vi "Writer Listen.vi"(8 "error in (no error)":errorcluster, 11 "TCP Writer in":refnum<class "TCP Writer.lvclass">) -> (0 "error out":errorcluster, 3 "TCP Writer out":refnum<class "TCP Writer.lvclass">)   [LabVIEW 2018, in "TCP Classes.lvlib" / "TCP Writer.lvclass"]
uses:
  TCP Writer.lvclass
  C:/Users/Jeff Tipps/Documents/DAQMan/source/Classes/TCP Server/Class TCP Connection/TCP Connection.lvclass
  C:/Program Files (x86)/National Instruments/LabVIEW 2018/vi.lib/ActorFramework/Actor/Actor.lvclass
  Class TCP Connection/TCP Connection.lvclass/TCP Connection.ctl
  TCP Writer.lvclass/TCP Writer.ctl
  Common/Controls/Waveform Header with Enbl.ctl
  Common/Controls/Waveform Header.ctl
  <vilib>/ActorFramework/Actor/Actor.lvclass/Actor.ctl
  <vilib>/ActorFramework/Message Enqueuer/Message Enqueuer.lvclass/Message Enqueuer.ctl
  Class TCP Connection/Read Connection.vi
  <vilib>/ActorFramework/Message Enqueuer/Init from Existing Queue.vi
  <vilib>/ActorFramework/Message Enqueuer/Enqueue.vi
  TCP Writer Messages/Writer Listen Msg/Writer Listen Msg.lvclass
  C:/Program Files (x86)/National Instruments/LabVIEW 2018/vi.lib/ActorFramework/Message/Message.lvclass
  Common/SubVIs/Conn Status Global.vi
  <vilib>/ActorFramework/Message Priority Queue/Priority Enqueue.vi
  <vilib>/ActorFramework/Message Enqueuer/Message Enqueuer.lvclass
  <vilib>/ActorFramework/Actor/Actor.lvclass
  Class TCP Connection/TCP Connection.lvclass
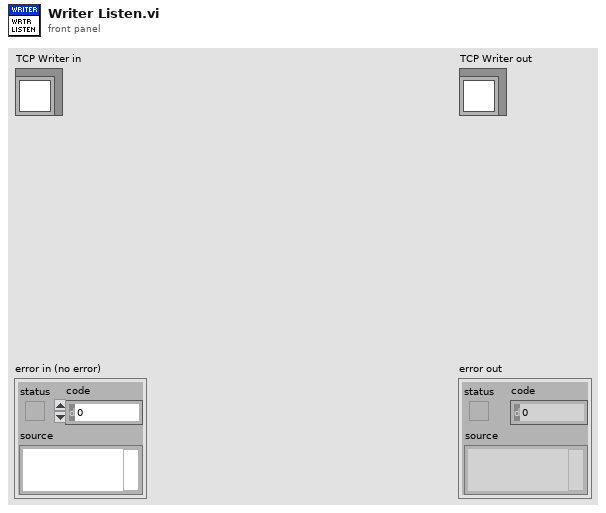
[diagram p1: front panel]
types:
  T1 = typedef "Waveform Header with Enbl.ctl" = cluster{"Send Wfm Hdr?":bool, "Wfm Header":T2}
  T2 = typedef "Waveform Header.ctl" = cluster{"dt":dbl, "attributes (str)":string[][]}
  T3 = enum16{"big-endian, network order", "native, host order", "little-endian"}
  T4 = typedef "stm_TCP Connection Info.ctl" = cluster{"connection ID":refnum<k5>, "Meta data":T5[]}
  T5 = typedef "stm_MetaDataElement.ctl" = string
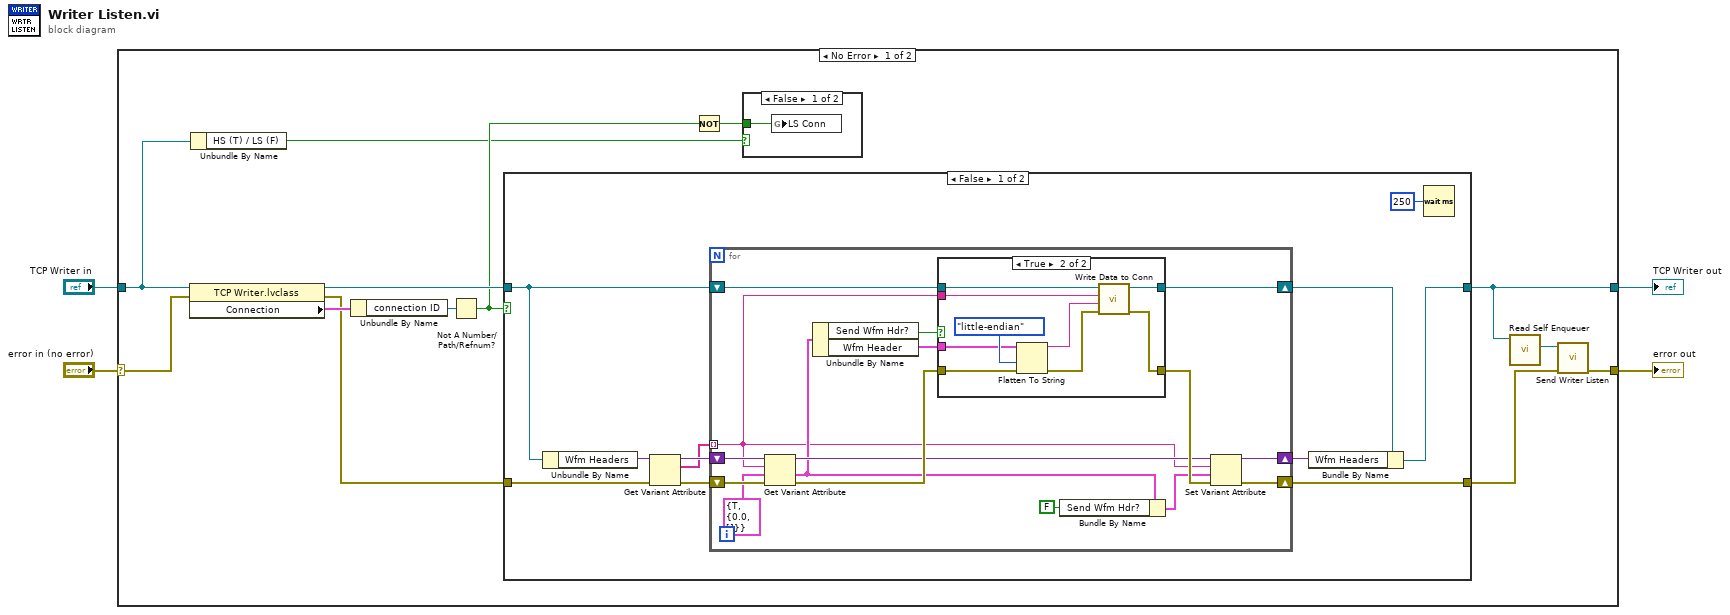
[diagram p0: block diagram]
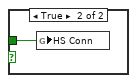
[diagram p2: hidden frame]
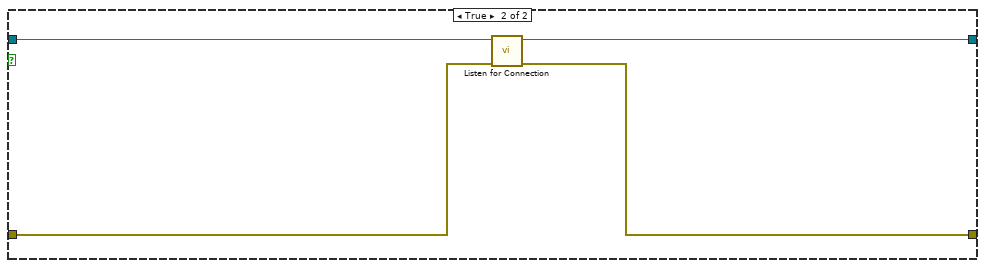
[diagram p4: hidden frame]
diagram:
  n1 = case shown="No Error" "error in (no error)" {
    selector: "error in (no error)" -> [w14 w63]
    tunnel: [w10 w63] -> w3
    tunnel: [w13 w62] -> w1
    tunnel: "TCP Writer in" -> [w6 w62]
    frame No Error {
      n2 = property class="TCP Writer.lvclass"(reference=w6, error in=w14) -> (reference out=w16:refnum<class "TCP Writer.lvclass">, error out=w5:errorcluster, "Connection"=w15:T4)
      n3 = Unbundle By Name(w6) -> ("HS (T) / LS (F)"=w7:bool)
      n4 = Unbundle By Name(w15) -> ("connection ID"=w17:refnum<k5>)
      n5 = Not A Number/Path/Refnum?(number/path/refnum=w17) -> (NaN/Path/Refnum?=w9:bool)
      n6 = case shown="False" w9 {
        tunnel: w16 -> [w27 w61]
        tunnel: [w20 w60] -> w13
        tunnel: [w29 w59] -> w12
        tunnel: w5 -> [w28 w58]
        frame False {
          n7 = Unbundle By Name(w27) -> ("Wfm Headers"=w23:variant)
          n8 = Get Variant Attribute(Variant=w23, error in=w28) -> (duplicate Variant=w26:variant, names=w25:string[], error out=w24:errorcluster)  [unwired: 2 in, 1 out]
          n9 = for {
            shift-right: [w45] -> w21
            shift-left: w27 -> [w46]
            shift-right: [w37] -> w29
            shift-left: w24 -> [w43]
            tunnel: w25 -> [w34] mode=indexing
            shift-right: [w31] -> w22
            shift-left: w26 -> [w44]
            n10 = Get Variant Attribute(Variant=w44, name=w34, default value (empty Variant)=T1 {"Send Wfm Hdr?"=TRUE, "Wfm Header"={"dt"=0.0, "attributes (str)"=[]}} ("Wfm Header with Enbl"), error in=w43) -> (duplicate Variant=w36:variant, value=w35:T1, error out=w40:errorcluster)  [unwired: 1 out]
            n11 = Unbundle By Name(w35) -> ("Send Wfm Hdr?"=w39:bool, "Wfm Header"=w41:T2)
            n12 = case shown="True" w39 {
              tunnel: [w47 w57] -> w38
              tunnel: w46 -> [w48 w56]
              tunnel: [w48 w55] -> w45
              tunnel: w34 -> [_ w51]
              tunnel: w41 -> [_ w50]
              tunnel: w40 -> [w47 w49]
              frame False {
              }
              frame True {
                n13 = Flatten To String(anything=w50, byte order (0:big-endian, network order)=T3."little-endian", error in (no error)=w49) -> (data string=w54:string, error out=w53:errorcluster)  [unwired: 1 in, 1 out]
                n14 = call "Write Data to Conn.vi"("error in (no error)"=w53, "Data"=w54, "MetaData"=w51, "TCP Connection in"=w56) -> ("error out"=w57:errorcluster, "TCP Connection out"=w55:refnum<class "TCP Writer.lvclass">)  [unwired: 6 in]
              }
            }
            n15 = Bundle By Name(cluster=w35, "Send Wfm Hdr?"=FALSE) -> (w32:T1)
            n16 = Set Variant Attribute(Variant=w36, name=w34, value=w32, error in=w38) -> (Variant out=w31:variant, error out=w37:errorcluster)  [unwired: 1 out]
          }
          n17 = Bundle By Name(cluster=w21, "Wfm Headers"=w22) -> (w20:refnum<class "TCP Writer.lvclass">)
          n18 = Wait (ms)(milliseconds to wait=u32 250) -> ()  [unwired: 1 out]
        }
        frame True {
          n19 = call-dynamic "Listen for Connection.vi"("error in (no error)"=w58, "TCP Writer in"=w61) -> ("error out"=w59:errorcluster, "TCP Writer out"=w60:refnum<class "TCP Writer.lvclass">)  [unwired: 7 in, 1 out]
        }
      }
      n20 = Not(x=w9) -> (.not. x?=w8:bool)
      n21 = case shown="False" w7 {
        tunnel: w8 -> [w18 w19]
        frame False {
          n22 = global write "Conn Status Global.vi" "LS Conn"(w18) -> ()
        }
        frame True {
          n23 = global write "Conn Status Global.vi" "HS Conn"(w19) -> ()
        }
      }
      n24 = call <vilib>:"Read Self Enqueuer.vi"("Actor"=w13) -> ("Self Enqueuer"=w11:refnum<class "Message Enqueuer.lvclass">)  [unwired: 10 in]
      n25 = call "Send Writer Listen.vi"("error in (no error)"=w12, "Message Enqueuer"=w11) -> ("error out"=w10:errorcluster)  [unwired: 8 in, 1 out]
    }
    frame Error {
    }
  }
  "error out" <- w3
  "TCP Writer out" <- w1
